vi "test.vi"() -> ()   [LabVIEW 2010]
panel:
  out "error out":errorcluster
  in  "stop":bool
  in  "DO Lines":bool[](array[boolean])=[FALSE, FALSE, FALSE, FALSE, FALSE, FALSE, FALSE, FALSE]
  in  "Lines to Write":u16(ring) items=["0 - 7", "8 - 15", "16 - 23"]
  in  "Device Name":tag
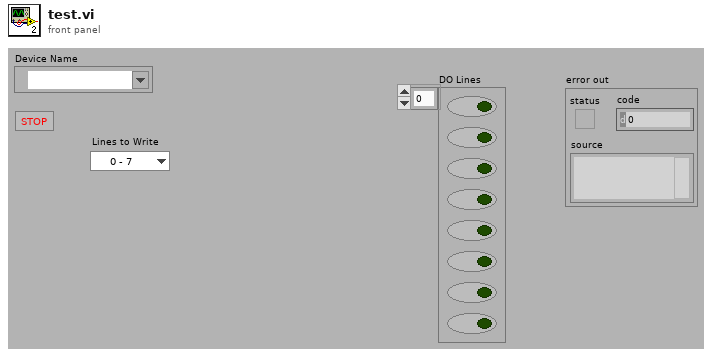
[diagram p1: front panel]
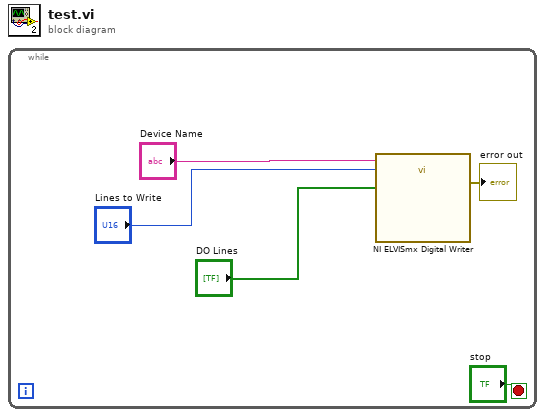
[diagram p0: block diagram]
diagram:
  n1 = while {
    stop <- "stop" stop-if-true
    n2 = call "NI ELVISmx Digital Writer"("Device Name"="Device Name", "Lines to Write"="Lines to Write", "DO Lines"="DO Lines") -> ("error out"=→"error out":errorcluster)  [unwired: 16 in]
  }
